vi "Setup For Triggered Images v4.2.vi"(4 "error in":errorcluster caption="error in (no error)", 5 "Timeout (ms)":u32=1000, 6 "Gain":dbl, 7 "Shutter speed":dbl, 8 "Camera Name":T3) -> (0 "Error out":errorcluster caption="error in (no error)", 1 "Session Out":T3, 2 "Height":u32, 3 "Width":u32)   [LabVIEW 2012]
doc: "The Grab and Attributes Setup VI acquires images continuously and displays the images in an image control using high-level acquisition VIs. The VI also modifes the camera attributes while acquiring images. A grab is appropriate for high-speed applications in which you need to process only one image at a time."
uses:
  <vilib>/userdefined/High Color/IMAQdx.ctl
  <vilib>/vision/driver/IMAQdx.llb/IMAQdx Attribute Type.ctl
  <vilib>/vision/driver/IMAQdx.llb/IMAQdx Attribute Visibility.ctl
  <vilib>/vision/driver/IMAQdx.llb/IMAQdx Acquisition Mode.ctl
  <vilib>/vision/driver/NI_Vision_Acquisition_Software.lvlib
  <resource>/objmgr/imaqdx.rc
panel:
  out "Attribute Information Array":T2(array[cluster])
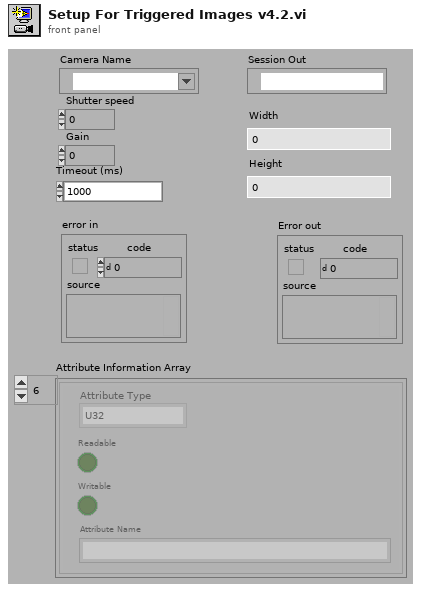
[diagram p1: front panel]
types:
  T1 = typedef "NI_Vision_Acquisition_Software.lvlib/IMAQdx Attribute Type.ctl" = enum32{"U32", "I64", "DBL", "String", "Enum", "Bool", "Command"}
  T2 = cluster{"Attribute Type":T1, "Readable":bool, "Writable":bool, "Attribute Name":string}[]
  T3 = typedef "IMAQdx.ctl" = refnum<k21>
  T4 = typedef "NI_Vision_Acquisition_Software.lvlib/IMAQdx Attribute Visibility.ctl" = enum32{"Simple", "Intermediate", "Advanced"}
  T5 = typedef "NI_Vision_Acquisition_Software.lvlib/IMAQdx Acquisition Mode.ctl" = enum32{"One Shot", "Continuous"}
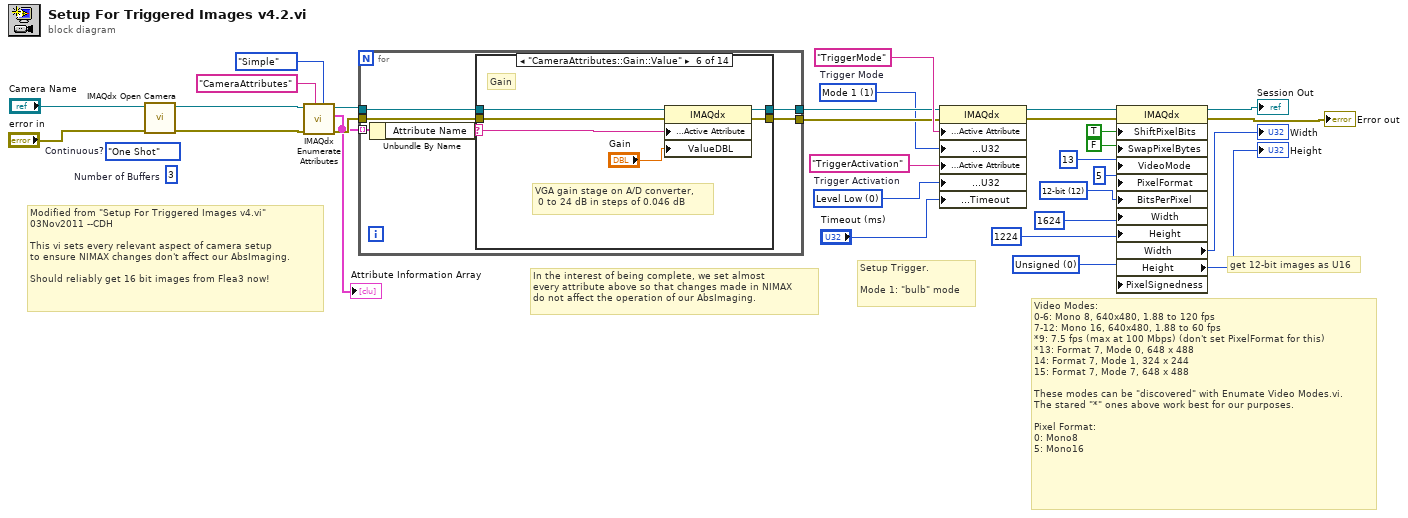
[diagram p0: block diagram]
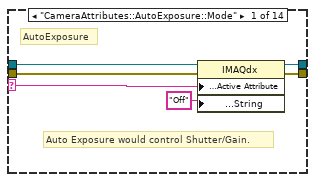
[diagram p2: hidden frame]
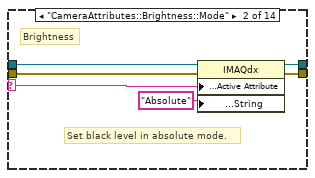
[diagram p3: hidden frame]
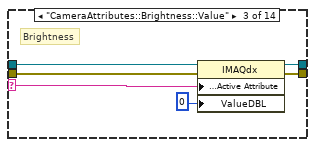
[diagram p4: hidden frame]
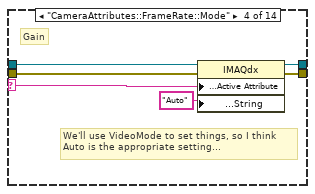
[diagram p5: hidden frame]
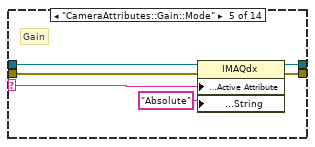
[diagram p6: hidden frame]
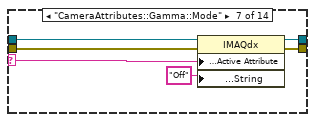
[diagram p7: hidden frame]
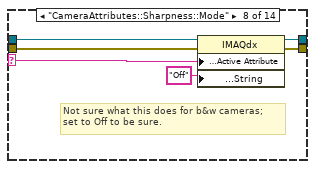
[diagram p8: hidden frame]
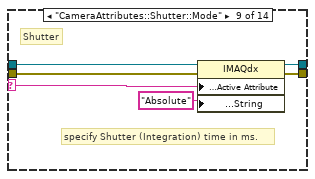
[diagram p9: hidden frame]
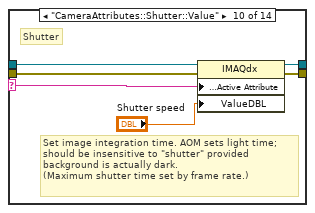
[diagram p10: hidden frame]
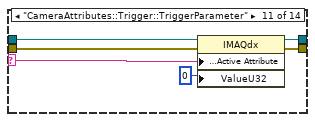
[diagram p11: hidden frame]
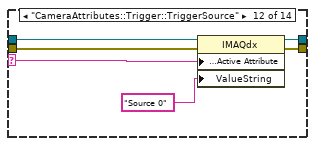
[diagram p12: hidden frame]
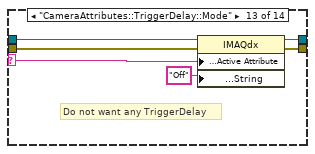
[diagram p13: hidden frame]
diagram:
  w6 = u32 0 items=["Unsigned", "Signed", "Use Hardware Value"] ("PixelSignedness")
  w9 = u32 12 items=["Use Hardware Value"=0, "10-bit"=10, "12-bit"=12, "14-bit"=14, "16-bit"=16] ("BitsPerPixel")
  w21 = u32 1 items=["Mode 0"=0, "Mode 1"=1, "Mode 3"=3, "Mode 14"=14, "Mode 15"=15, "Off"=16]  # Trigger Mode
  w20 = u32 0 items=["Level Low", "Level High"]  # Trigger Activation
  (unwired) u32 3  # Number of Buffers
  (unwired) IMAQdx_Acquisition_Mode."One Shot"  # Continuous?
  # "Modified from \"Setup For Triggered Images v4.vi\"\n03Nov2011 --CDH\n\nThis vi sets every relevant aspect of camera setup\nto ensure NIMAX changes don't affect our AbsImaging.\n\nShould reliably get 16 bit images from Flea3 now!"
  # "get 12-bit images as U16"
  # "In the interest of being complete, we set almost\nevery attribute above so that changes made in NIMAX\ndo not affect the operation of our AbsImaging."
  # "Video Modes:\n0-6: Mono 8, 640x480, 1.88 to 120 fps\n7-12: Mono 16, 640x480, 1.88 to 60 fps\n*9: 7.5 fps (max at 100 Mbps) (don't set PixelFormat for this)\n*13: Format 7, Mode 0, 648 x 488\n14: Format 7, Mode 1, 324 x 244\n15: Format 7, Mode 7, 648 x 488 \n\nThese modes can be \"discovered\" with Enumate Video Modes.vi.\nThe stared \"*\" ones above work best for our purposes.\n\nPixel Format:\n0: Mono8\n5: Mono16"
  # "Setup Trigger.\n\nMode 1: \"bulb\" mode"
  n1 = call <vilib>:"IMAQdx Open Camera.vi"("error in"="error in", "Session In"="Camera Name") -> ("error out"=w12:errorcluster, "Session Out"=w13:T3)  [unwired: 1 in, 7 out]
  n2 = call <vilib>:"IMAQdx Enumerate Attributes.vi"("Visibility"=IMAQdx_Attribute_Visibility."Simple", "Root"="CameraAttributes", "error in"=w12, "Session In"=w13) -> ("error out"=w30:errorcluster, "Attribute Information Array"=w26:T2, "Session Out"=w29:T3)  [unwired: 5 out]
  "Attribute Information Array" <- w26
  n3 = for {
    tunnel: w26 -> [w36] mode=indexing
    tunnel: w29 -> [w35]
    tunnel: w30 -> [w34]
    tunnel: [w32] -> w23
    tunnel: [w31] -> w22
    n4 = Unbundle By Name(w36) -> ("Attribute Name"=w33:string)
    n5 = case shown="\"CameraAttributes::Gain::Value\"" w33 {
      selector: w33 -> [w38 w44 w50 w56 w62 w68 w74 w80 w86 w92 w98 w104 w110 _]
      tunnel: w35 -> [w42 w48 w54 w60 w66 w72 w78 w84 w90 w96 w102 w108 w114 w116]
      tunnel: w34 -> [w41 w47 w53 w59 w65 w71 w77 w83 w89 w95 w101 w107 w113 w115]
      tunnel: [w40 w46 w52 w58 w64 w70 w76 w82 w88 w94 w100 w106 w112 w116] -> w32
      tunnel: [w39 w45 w51 w57 w63 w69 w75 w81 w87 w93 w99 w105 w111 w115] -> w31
      frame "CameraAttributes::AutoExposure::Mode" {
        # "Auto Exposure would control Shutter/Gain."
        # "AutoExposure"
        n6 = property class="IMAQdx"(reference=w42, error in=w41, "Camera Attributes:Active Attribute"=w38, "Camera Attributes:Value:String"="Off" ("ValueString")) -> (reference out=w40:T3, error out=w39:errorcluster)
      }
      frame "CameraAttributes::Brightness::Mode" {
        # "Set black level in absolute mode."
        # "Brightness"
        n7 = property class="IMAQdx"(reference=w48, error in=w47, "Camera Attributes:Active Attribute"=w44, "Camera Attributes:Value:String"="Absolute" ("ValueString")) -> (reference out=w46:T3, error out=w45:errorcluster)
      }
      frame "CameraAttributes::Brightness::Value" {
        # "Brightness"
        n8 = property class="IMAQdx"(reference=w54, error in=w53, "Camera Attributes:Active Attribute"=w50, "ValueDBL"=0) -> (reference out=w52:T3, error out=w51:errorcluster)
      }
      frame "CameraAttributes::FrameRate::Mode" {
        # "We'll use VideoMode to set things, so I think\nAuto is the appropriate setting..."
        # "Gain"
        n9 = property class="IMAQdx"(reference=w60, error in=w59, "Camera Attributes:Active Attribute"=w56, "Camera Attributes:Value:String"="Auto" ("ValueString")) -> (reference out=w58:T3, error out=w57:errorcluster)
      }
      frame "CameraAttributes::Gain::Mode" {
        # "Gain"
        n10 = property class="IMAQdx"(reference=w66, error in=w65, "Camera Attributes:Active Attribute"=w62, "Camera Attributes:Value:String"="Absolute" ("ValueString")) -> (reference out=w64:T3, error out=w63:errorcluster)
      }
      frame "CameraAttributes::Gain::Value" {
        # "VGA gain stage on A/D converter,\n 0 to 24 dB in steps of 0.046 dB"
        # "Gain"
        n11 = property class="IMAQdx"(reference=w72, error in=w71, "Camera Attributes:Active Attribute"=w68, "ValueDBL"="Gain") -> (reference out=w70:T3, error out=w69:errorcluster)
      }
      frame "CameraAttributes::Gamma::Mode" {
        n12 = property class="IMAQdx"(reference=w78, error in=w77, "Camera Attributes:Active Attribute"=w74, "Camera Attributes:Value:String"="Off" ("ValueString")) -> (reference out=w76:T3, error out=w75:errorcluster)
      }
      frame "CameraAttributes::Sharpness::Mode" {
        # "Not sure what this does for b&w cameras;\nset to Off to be sure."
        n13 = property class="IMAQdx"(reference=w84, error in=w83, "Camera Attributes:Active Attribute"=w80, "Camera Attributes:Value:String"="Off" ("ValueString")) -> (reference out=w82:T3, error out=w81:errorcluster)
      }
      frame "CameraAttributes::Shutter::Mode" {
        # "specify Shutter (Integration) time in ms."
        # "Shutter"
        n14 = property class="IMAQdx"(reference=w90, error in=w89, "Camera Attributes:Active Attribute"=w86, "Camera Attributes:Value:String"="Absolute" ("ValueString")) -> (reference out=w88:T3, error out=w87:errorcluster)
      }
      frame "CameraAttributes::Shutter::Value" {
        # "Set image integration time. AOM sets light time;\nshould be insensitive to \"shutter\" provided \nbackground is actually dark.\n(Maximum shutter time set by frame rate.)"
        # "Shutter"
        n15 = property class="IMAQdx"(reference=w96, error in=w95, "Camera Attributes:Active Attribute"=w92, "ValueDBL"="Shutter speed") -> (reference out=w94:T3, error out=w93:errorcluster)
      }
      frame "CameraAttributes::Trigger::TriggerParameter" {
        n16 = property class="IMAQdx"(reference=w102, error in=w101, "Camera Attributes:Active Attribute"=w98, "ValueU32"=u32 0) -> (reference out=w100:T3, error out=w99:errorcluster)
      }
      frame "CameraAttributes::Trigger::TriggerSource" {
        n17 = property class="IMAQdx"(reference=w108, error in=w107, "Camera Attributes:Active Attribute"=w104, "ValueString"="Source 0") -> (reference out=w106:T3, error out=w105:errorcluster)
      }
      frame "CameraAttributes::TriggerDelay::Mode" {
        # "Do not want any TriggerDelay"
        n18 = property class="IMAQdx"(reference=w114, error in=w113, "Camera Attributes:Active Attribute"=w110, "Camera Attributes:Value:String"="Off" ("ValueString")) -> (reference out=w112:T3, error out=w111:errorcluster)
      }
      frame Default {
      }
    }
  }
  n19 = property class="IMAQdx"(reference=w23, error in=w22, "Camera Attributes:Active Attribute"="TriggerMode" ("ActiveAttribute"), "Camera Attributes:Value:U32"=w21, "Camera Attributes:Active Attribute"="TriggerActivation" ("ActiveAttribute"), "Camera Attributes:Value:U32"=w20, "Acquisition Attributes:Timeout"="Timeout (ms)") -> (reference out=w18:T3, error out=w17:errorcluster)
  n20 = property class="IMAQdx"(reference=w18, error in=w17, "ShiftPixelBits"=TRUE, "SwapPixelBytes"=FALSE, "VideoMode"=u32 13, "PixelFormat"=u32 5, "BitsPerPixel"=w9, "Width"=u32 1624, "Height"=u32 1224, "PixelSignedness"=w6) -> (reference out=→"Session Out":T3, error out=→"Error out":errorcluster, "Width"=→"Width":u32, "Height"=→"Height":u32)
